vi "Advanced Counter Sub.vi"(4 "Reset Counter":bool, 5 "Init Counter Value":u32, 6 "Enable HW Gate":bool, 7 "Ticks to Filter":u32, 8 "Count Direction":enum16{"Up", "Down"}(ring), 9 "Edge":T1(ring), 10 "Gate Signal":bool, 11 "Input Signal":bool) -> (1 "Counter Reset?":bool, 3 "Counter Out":u32)   [LabVIEW 2020]
uses:
  <vilib>/rvi/Emulation/niFpgaSctlEmulationGetInTimedLoop.vi
  <vilib>/rvi/Emulation/niFpgaProcessEmulError.vi
panel:
  out "Input Signal (Out)":bool
  out "Output Filtered Signal":bool
  out "Bucket Out":u32
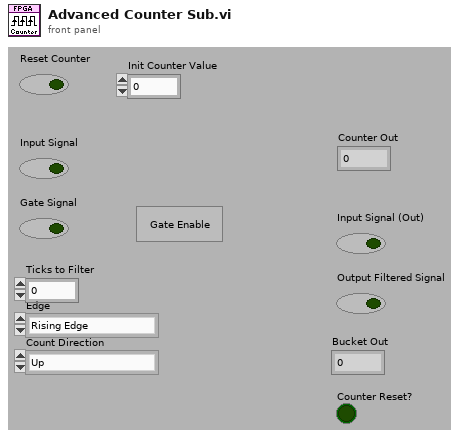
[diagram p1: front panel]
types:
  T1 = enum16{"Rising Edge", "Falling Edge", "Rising AND Falling Edges"}
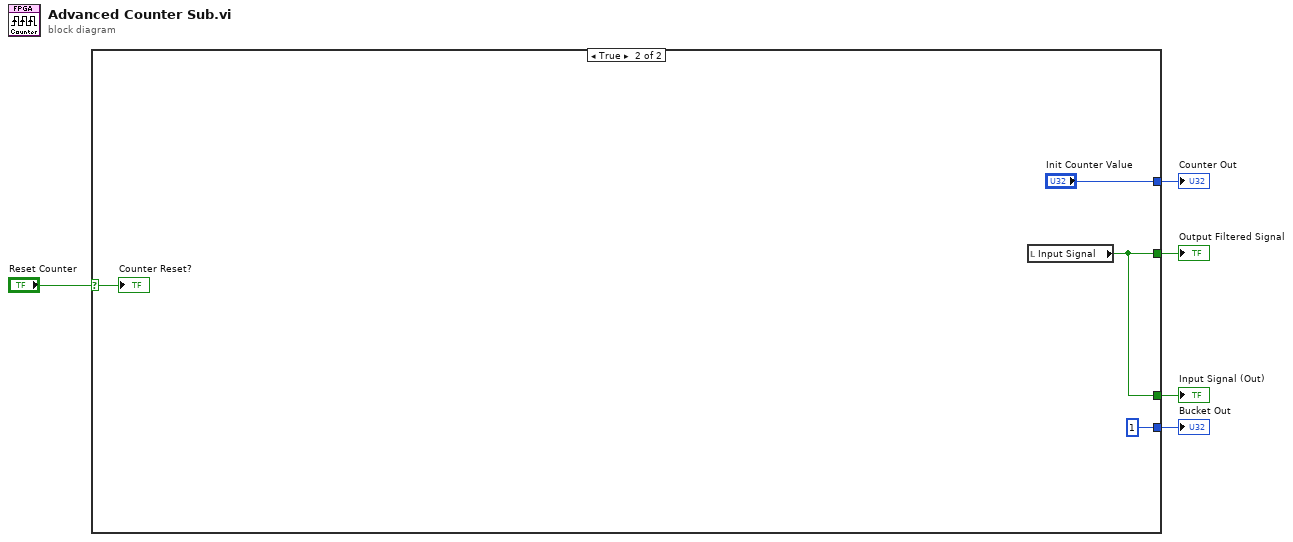
[diagram p0: block diagram]
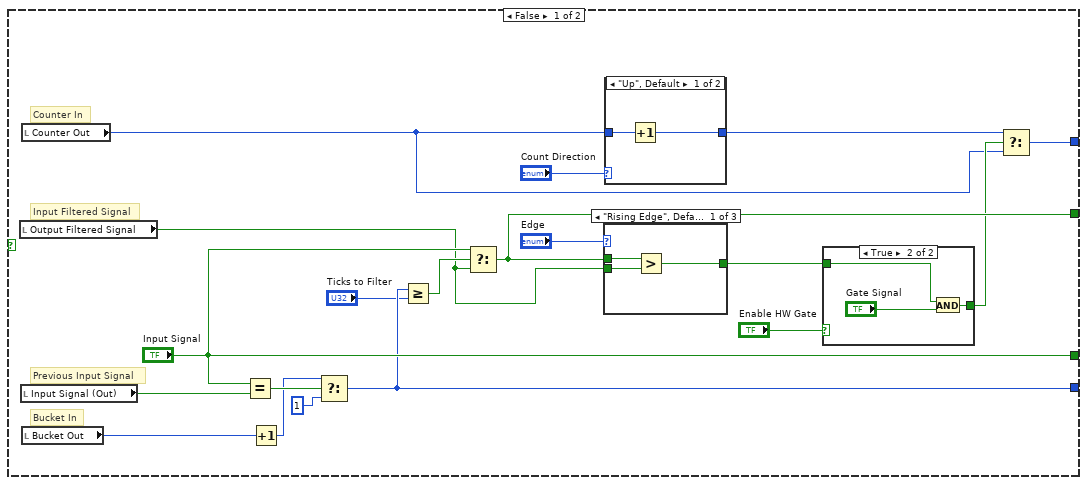
[diagram p2: hidden frame]
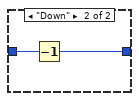
[diagram p4: hidden frame]
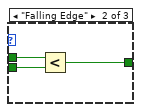
[diagram p5: hidden frame]
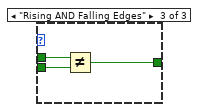
[diagram p6: hidden frame]
diagram:
  n1 = case shown="True" "Reset Counter" {
    selector: "Reset Counter" -> [_ w45]
    tunnel: ["Input Signal" w42] -> w4
    tunnel: [w23 "Init Counter Value"] -> w3
    tunnel: [w22 u32 1 ("Counter Out")] -> w2
    tunnel: [w21 w42] -> w1
    frame False {
      # "Bucket In"
      # "Counter In"
      # "Input Filtered Signal"
      # "Previous Input Signal"
      n2 = local read "Output Filtered Signal"() -> (w7:bool)
      n3 = local read "Input Signal (Out)"() -> (w8:bool)
      n4 = local read "Counter Out"() -> (w6:u32)
      n5 = local read "Bucket Out"() -> (w9:u32)
      n6 = Equal?(x="Input Signal", y=w8) -> (x = y?=w20:bool)
      n7 = Increment(x=w9) -> (x+1=w19:u32)
      n8 = Select(t=w19, s=w20, f=u32 1) -> (s? t:f=w22:u32)
      n9 = Greater Or Equal?(x=w22, y="Ticks to Filter") -> (x >= y?=w16:bool)
      n10 = Select(t="Input Signal", s=w16, f=w7) -> (s? t:f=w21:bool)
      n11 = case shown="\"Rising Edge\", Default" "Edge" {
        tunnel: w21 -> [w35 w38 w41]
        tunnel: [w34 w37 w40] -> w13
        tunnel: w7 -> [w33 w36 w39]
        frame "Rising Edge", Default {
          n12 = Greater?(x=w35, y=w33) -> (0:w34:bool)
        }
        frame "Falling Edge" {
          n13 = Less?(x=w38, y=w36) -> (x < y?=w37:bool)
        }
        frame "Rising AND Falling Edges" {
          n14 = Not Equal?(x=w41, y=w39) -> (x != y?=w40:bool)
        }
      }
      n15 = case shown="\"Up\", Default" "Count Direction" {
        tunnel: w6 -> [w30 w32]
        tunnel: [w29 w31] -> w15
        frame "Up", Default {
          n16 = Increment(x=w30) -> (x+1=w29:u32)
        }
        frame "Down" {
          n17 = Decrement(x=w32) -> (x-1=w31:u32)
        }
      }
      n18 = case shown="True" "Enable HW Gate" {
        tunnel: w13 -> [w25 w28]
        tunnel: [w25 w27] -> w12
        frame False {
        }
        frame True {
          n19 = And(x=w28, y="Gate Signal") -> (x .and. y?=w27:bool)
        }
      }
      n20 = Select(t=w15, s=w12, f=w6) -> (s? t:f=w23:u32)
    }
    frame True {
      n21 = local read "Input Signal"() -> (w42:bool)
      "Counter Reset?" <- w45
    }
  }
  "Input Signal (Out)" <- w4
  "Counter Out" <- w3
  "Bucket Out" <- w2
  "Output Filtered Signal" <- w1
